vi "Coord list setup unbundler-STRING.vi"(8 "error in (no error)":errorcluster, 9 "Keys Array":T1, 10 "Section name":string, 11 "User profile ini file ref":T2) -> (0 "error out":errorcluster, 3 "User profile ini file ref":T2)   [LabVIEW 2020]
uses:
  <vilib>/Utility/config.llb/Config Data RefNum.ctl
  Typedefs/Ini file interface (String).ctl
  User Interface/Windows/Coordinates list window/Globals/Coord window-Globals.vi
  <vilib>/Utility/config.llb/NI_LVConfig.lvlib
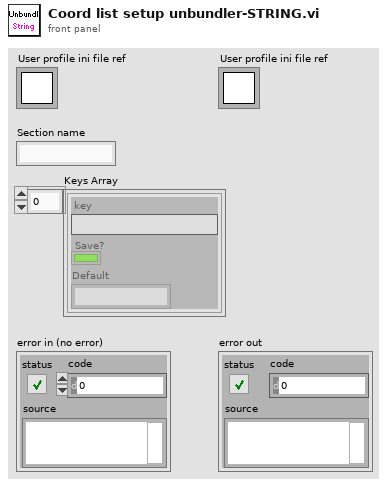
[diagram p1: front panel]
types:
  T1 = typedef "Ini file interface (String).ctl" = cluster{"key":string, "Save?":bool, "Default":string}[]
  T2 = typedef "NI_LVConfig.lvlib/Config Data RefNum.ctl" = refnum<k1>
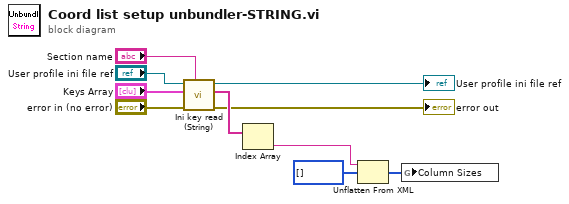
[diagram p0: block diagram]
diagram:
  n1 = call "Ini key read (String).vi"("Section name"="Section name", "error in (no error)"="error in (no error)", "Keys setup"="Keys Array", "Ini file ref in"="User profile ini file ref") -> ("error out"=→"error out":errorcluster, "Value read/used"=w3:string[], "Ini file ref"=→"User profile ini file ref":T2)  [unwired: 5 in]
  n2 = Index Array(array=w3) -> (element=w10:string)  [unwired: 1 in]
  n3 = Unflatten From XML(xml string=w10, type=u32[] [] ("Column Sizes")) -> (value=w8:u32[])  [unwired: 1 in, 1 out]
  n4 = global write "Coord window-Globals.vi" "Column Sizes"(w8) -> ()
